vi "Drive Controller.vi"(8 "error in":errorcluster) -> ()   [LabVIEW 2020]
doc: "This VI executes continuously carrying out the current operation and responding to updates or new operation requests. It will often contain the timing or control code that is difficult to place directly in TeleOp. This VI generally opens all sensors and motors and isolates the rest of the robot code from knowing implementation details of how the operations are carried out."
uses:
  <vilib>/Rock Robotics/WPI/Framework/Completion Status.ctl
  Drive Setpoints.ctl
  Drive Operations.ctl
  <vilib>/Rock Robotics/WPI/SafetyOutput/WPI_SafetyOutputConfigMenu.ctl
  <vilib>/Rock Robotics/WPI/ThirdParty/REV Robotics/REVLib/Typedef/Spark MAX Motor Type.ctl
  <vilib>/Rock Robotics/WPI/ThirdParty/REV Robotics/REVLib/Typedef/Spark MAX Idle Mode.ctl
  <vilib>/Rock Robotics/WPI/RobotDrive/WPI_RobotDriveOpen2MotorWithExistingMotors.vi
  <vilib>/Rock Robotics/Network Tables/NT Write Numeric Array.vi
panel:
  in  "Interactive Values":T1
  in  "Buttons":cluster{"Execute Cmd":bool, "Abort Cmd":bool}
  out "Command Timing":cluster{"Start Time (ms)":u32, "Iterations":i32}
  out "Status":T3
  out "Setpoints":T4(graph)
  out "Current\nCmd":string
  # "Tip: The graph shows the motor setpoints. It may also be helpful to observe inputs and sensor values.\nYou may also want to display tuning or debugging controls."
  # "Interactive Command: You may fill in the settings for a command\nand schedule it with the Execute button. You can observe and abort\nany command while fine tuning the code for the controller."
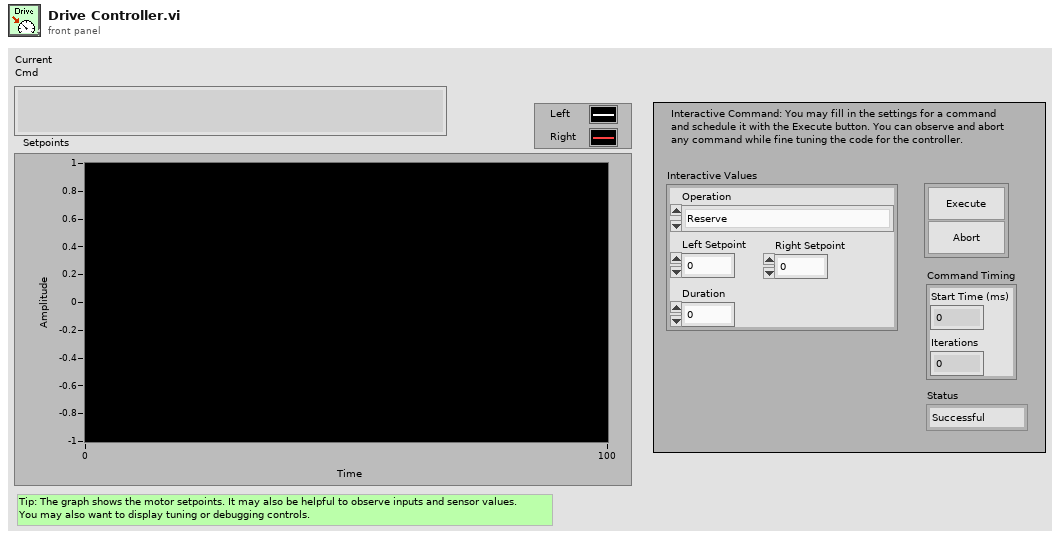
[diagram p1: front panel]
types:
  T1 = typedef "Drive Setpoints.ctl" = cluster{"Operation":T2, "Left Setpoint":dbl, "Right Setpoint":dbl, "Duration":dbl}
  T2 = typedef "Drive Operations.ctl" = enum16{"Reserve", "Read Current", "Immediate", "Drive for Time", "Drive for Distance"}
  T3 = typedef "Completion Status.ctl" = enum16{"Successful", "Aborted", "Incomplete"}
  T4 = cluster{"Left Setpoint":dbl, "Right Setpoint":dbl}
  T5 = typedef "Spark MAX Idle Mode.ctl" = enum16{"Coast", "Brake"}
  T6 = typedef "Spark MAX Motor Type.ctl" = enum16{"Brushed", "Brushless"}
  T7 = typedef "WPI_SafetyOutputConfigMenu.ctl" = enum16{"Enable", "Disable"}
  T8 = typedef "WPI_MotorControlDeviceRef.ctl" = cluster{"DeviceStatus":errorcluster, "Type":T9, "PWM":cluster{"PWM Channel":T10, "DeadBand":T11}, "CAN":cluster{"Device Number":u8, "SetOutput VI Ref":variant, "GetOutput VI Ref":variant, "Enable VI Ref":variant, "Disable VI Ref":variant, "Data":variant}, "Invert":bool, "DIO PWM":cluster{"PWM \"Enable\" Channel":T10, "DIOChannel":T12, "PWM Rate":dbl}}
  T9 = typedef "WPI_MotorControlType.ctl" = enum16{"PWM", "CAN", "DIO PWM"}
  T10 = typedef "FPGA_DIOPWMChannel.ctl" = enum8{"PWM 0", "PWM 1", "PWM 2", "PWM 3", "PWM 4", "PWM 5", "PWM 6", "PWM 7", "PWM 8", "PWM 9", "PWM MXP 0", "PWM MXP 1", "PWM MXP 2", "PWM MXP 3", "PWM MXP 4", "PWM MXP 5", "PWM MXP 6", "PWM MXP 7", "PWM MXP 8", "PWM MXP 9", "Invalid"}
  T11 = typedef "WPI_PWMDeadband.ctl" = cluster{"Name":string, "maxPositivePwm":i32, "minPositivePwm":i32, "centerPwm":i32, "maxNegativePwm":i32, "minNegativePwm":i32, "angularRange":u16}
  T12 = typedef "FPGA_DIOChannel.ctl" = enum8{"DIO 0", "DIO 1", "DIO 2", "DIO 3", "DIO 4", "DIO 5", "DIO 6", "DIO 7", "DIO 8", "DIO 9", "DIO MXP 0", "DIO MXP 1", "DIO MXP 2", "DIO MXP 3", "DIO MXP 4", "DIO MXP 5", "DIO MXP 6", "DIO MXP 7", "DIO MXP 8", "DIO MXP 9", "DIO MXP 10", "DIO MXP 11", "DIO MXP 12", "DIO MXP 13", "DIO MXP 14", "DIO MXP 15", "SPI Port CS1", "SPI Port CS2", "SPI Port CS3", "SPI Port MISO", "SPI Port MOSI", "Invalid"}
  T13 = typedef "WPI_RobotDriveDevRef.ctl" = cluster{"DevStatus":errorcluster, "Motors[]":T8[], "Square Inputs":bool, "Max Output":dbl}
  T14 = typedef "Command Status Info.ctl" = cluster{"Name":string, "Status":T3, "notifier out":T15}
  T15 = typedef "Completion Notifier.ctl" = refnum<notifier>
  T16 = cluster{"SubSystem Data":T1, cluster{"Start Time (ms)":u32, "Iterations":i32}, cluster{"Command Info":T14, "Description":string, "Default Command":T1, "queue out":refnum<queue>, "Subsystem Name":string}}
  T17 = cluster{"SubSystem Data":T1, cluster{"Start Time (ms)":u32, "Iterations":i32}, "Default Command Arguments":cluster{"Command Info":T14, "Description":string, "Default Command":T1, "queue out":refnum<queue>, "Subsystem Name":string}}
  T18 = cluster{"Don't move motors while reserved":dbl, "Don't move motors while reserved":dbl}
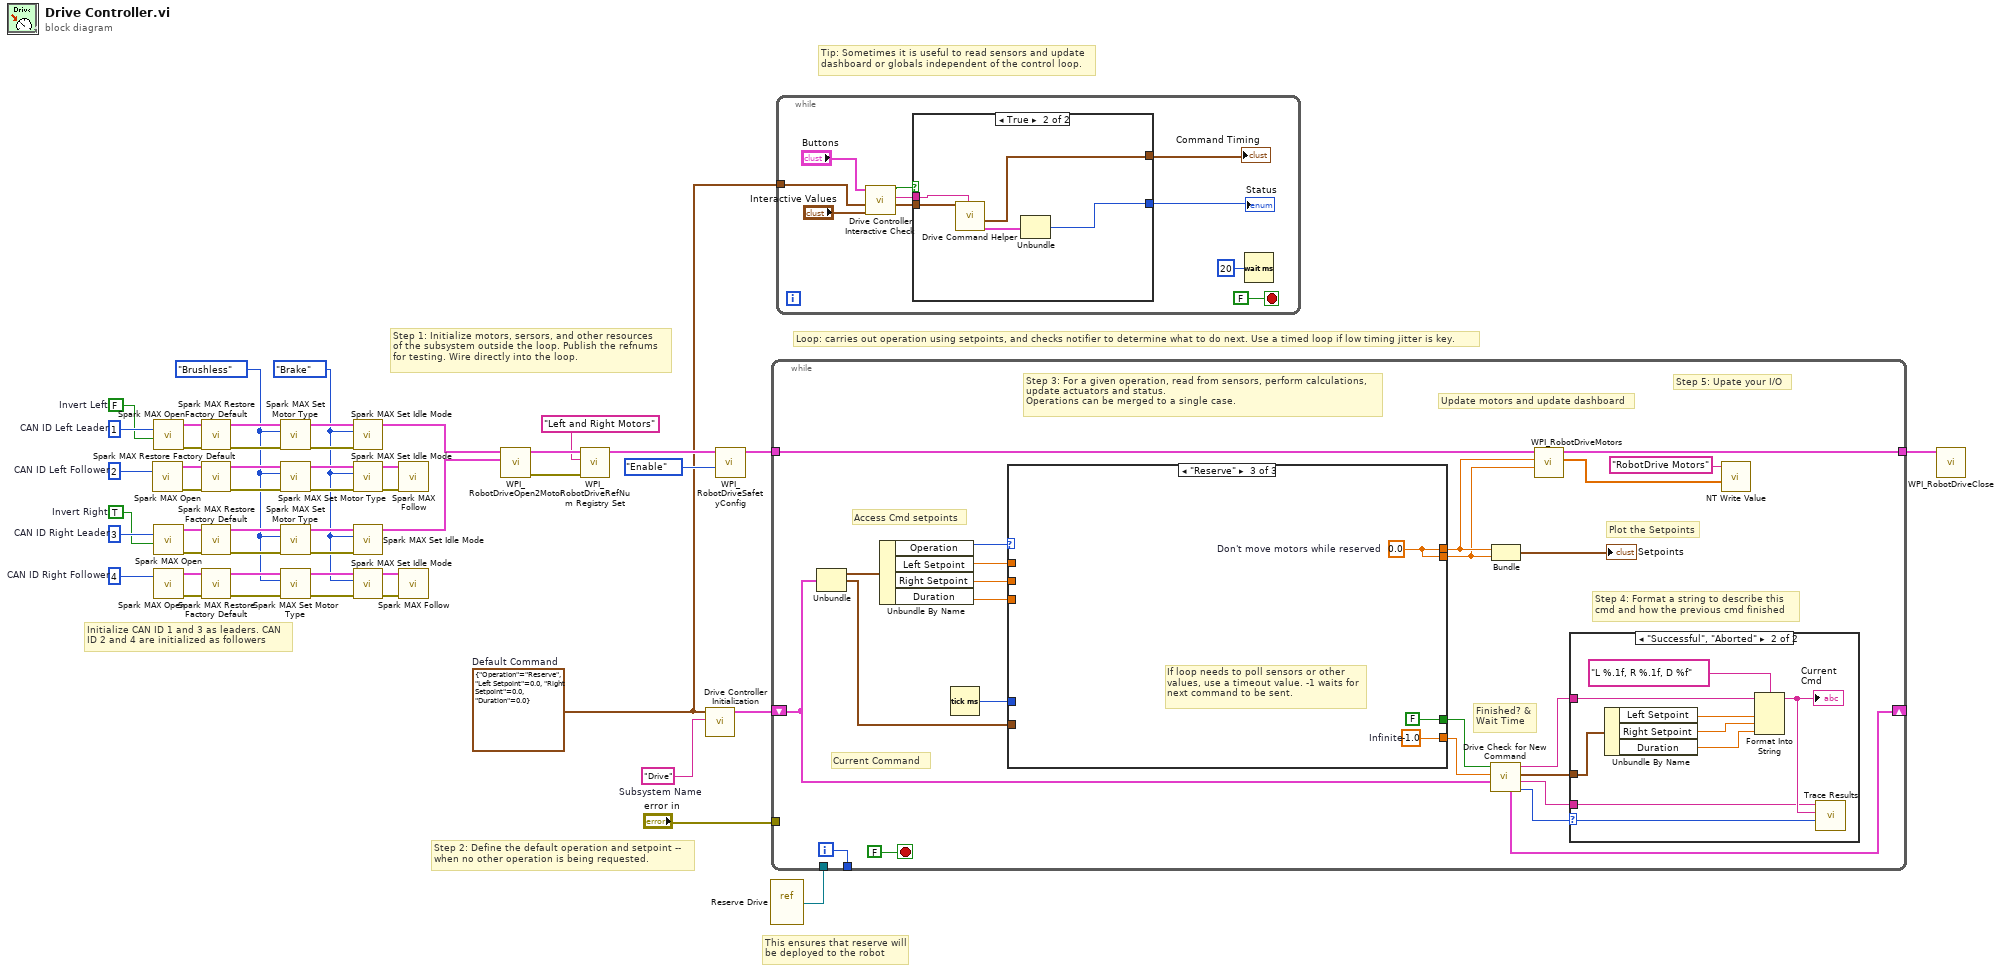
[diagram p0: block diagram]
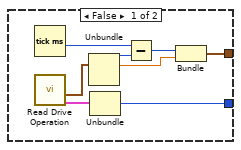
[diagram p2: hidden frame]
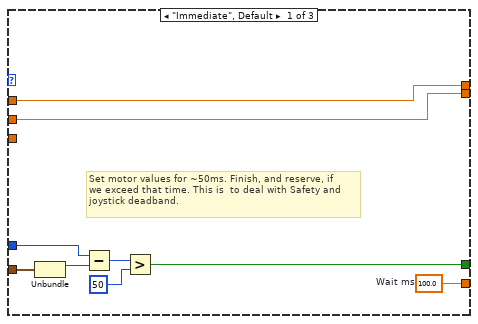
[diagram p4: hidden frame]
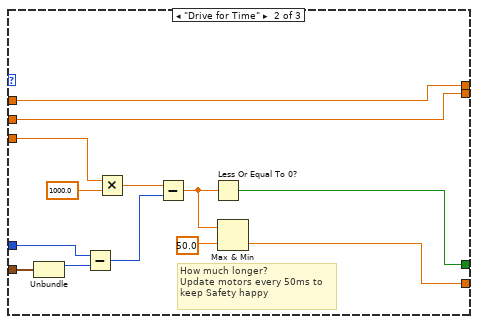
[diagram p5: hidden frame]
diagram:
  w8 = Spark_MAX_Idle_Mode."Brake" ("Idle Mode")
  w17 = Spark_MAX_Motor_Type."Brushless" ("Motor Type")
  w34 = FALSE  # Invert Left
  w35 = TRUE  # Invert Right
  w37 = u8 3  # CAN ID Right Leader
  w36 = u8 4  # CAN ID Right Follower
  w38 = u8 1  # CAN ID Left Leader
  w39 = u8 2  # CAN ID Left Follower
  w40 = T1 {"Operation"=enum."Reserve", "Left Setpoint"=0.0, "Right Setpoint"=0.0, "Duration"=0.0}  # Default Command
  w50 = "Drive"  # Subsystem Name
  # "Initialize CAN ID 1 and 3 as leaders. CAN \nID 2 and 4 are initialized as followers"
  # "This ensures that reserve will\nbe deployed to the robot"
  # "Tip: Sometimes it is useful to read sensors and update\ndashboard or globals independent of the control loop."
  # "Step 2: Define the default operation and setpoint --\nwhen no other operation is being requested."
  # "Step 1: Initialize motors, sersors, and other resources\nof the subsystem outside the loop. Publish the refnums\nfor testing. Wire directly into the loop."
  # "Loop: carries out operation using setpoints, and checks notifier to determine what to do next. Use a timed loop if low timing jitter is key."
  n1 = call <vilib>:"Spark MAX Open.vi"("Device Number"=w39) -> ("error out"=w31:errorcluster, "MotorControlDeviceRef"=w30:T8)  [unwired: 9 in]
  n2 = call <vilib>:"Spark MAX Open.vi"("Invert"=w34, "Device Number"=w38) -> ("error out"=w33:errorcluster, "MotorControlDeviceRef"=w32:T8)  [unwired: 8 in]
  n3 = call <vilib>:"Spark MAX Open.vi"("Invert"=w35, "Device Number"=w37) -> ("error out"=w29:errorcluster, "MotorControlDeviceRef"=w28:T8)  [unwired: 8 in]
  n4 = call <vilib>:"Spark MAX Open.vi"("Device Number"=w36) -> ("error out"=w27:errorcluster, "MotorControlDeviceRef"=w26:T8)  [unwired: 9 in]
  n5 = call <vilib>:"Spark MAX Restore Factory Default.vi"("error in"=w33, "MotorControlDeviceRef"=w32) -> ("error out"=w25:errorcluster, "MotorControlDeviceRef"=w24:T8)  [unwired: 8 in]
  n6 = call <vilib>:"Spark MAX Restore Factory Default.vi"("error in"=w31, "MotorControlDeviceRef"=w30) -> ("error out"=w23:errorcluster, "MotorControlDeviceRef"=w22:T8)  [unwired: 8 in]
  n7 = call <vilib>:"Spark MAX Restore Factory Default.vi"("error in"=w29, "MotorControlDeviceRef"=w28) -> ("error out"=w21:errorcluster, "MotorControlDeviceRef"=w20:T8)  [unwired: 8 in]
  n8 = call <vilib>:"Spark MAX Restore Factory Default.vi"("error in"=w27, "MotorControlDeviceRef"=w26) -> ("error out"=w19:errorcluster, "MotorControlDeviceRef"=w18:T8)  [unwired: 8 in]
  n9 = call <vilib>:"Spark MAX Set Motor Type.vi"("error in (no error)"=w25, "Motor Type"=w17, "MotorControlDevRef"=w24) -> ("error out"=w16:errorcluster, "MotorControlDeviceRef"=w15:T8)  [unwired: 7 in]
  n10 = call <vilib>:"Spark MAX Set Motor Type.vi"("error in (no error)"=w23, "Motor Type"=w17, "MotorControlDevRef"=w22) -> ("error out"=w14:errorcluster, "MotorControlDeviceRef"=w13:T8)  [unwired: 7 in]
  n11 = call <vilib>:"Spark MAX Set Motor Type.vi"("error in (no error)"=w21, "Motor Type"=w17, "MotorControlDevRef"=w20) -> ("error out"=w12:errorcluster, "MotorControlDeviceRef"=w11:T8)  [unwired: 7 in]
  n12 = call <vilib>:"Spark MAX Set Motor Type.vi"("error in (no error)"=w19, "Motor Type"=w17, "MotorControlDevRef"=w18) -> ("error out"=w10:errorcluster, "MotorControlDeviceRef"=w9:T8)  [unwired: 7 in]
  n13 = call <vilib>:"Spark MAX Set Idle Mode.vi"("error in (no error)"=w16, "Idle Mode"=w8, "MotorControlDeviceRef in"=w15) -> ("MotorControlDeviceRef out"=w3:T8)  [unwired: 7 in, 1 out]
  n14 = call <vilib>:"Spark MAX Set Idle Mode.vi"("error in (no error)"=w14, "Idle Mode"=w8, "MotorControlDeviceRef in"=w13) -> ("error out"=w7:errorcluster, "MotorControlDeviceRef out"=w6:T8)  [unwired: 7 in]
  n15 = call <vilib>:"Spark MAX Set Idle Mode.vi"("error in (no error)"=w12, "Idle Mode"=w8, "MotorControlDeviceRef in"=w11) -> ("MotorControlDeviceRef out"=w2:T8)  [unwired: 7 in, 1 out]
  n16 = call <vilib>:"Spark MAX Set Idle Mode.vi"("error in (no error)"=w10, "Idle Mode"=w8, "MotorControlDeviceRef in"=w9) -> ("error out"=w5:errorcluster, "MotorControlDeviceRef out"=w4:T8)  [unwired: 7 in]
  n17 = call <vilib>:"Spark MAX Follow.vi"("error in (no error)"=w7, "MotorControlDeviceRef"=w6) -> ()  [unwired: 8 in, 2 out]
  n18 = call <vilib>:"Spark MAX Follow.vi"("error in (no error)"=w5, "MotorControlDeviceRef"=w4) -> ()  [unwired: 8 in, 2 out]
  n19 = call-poly <vilib>:"WPI_RobotDriveOpen2Motor.vi"("Right Motor Dev Ref"=w2, "Left Motor Dev Ref"=w3) -> ("error out"=w47:errorcluster, "RobotDriveDevRef"=w49:T13)  [unwired: 3 in, 5 out]
  n20 = call <vilib>:"WPI_RobotDriveRefNum Registry Set.vi"("error in (no error)"=w47, "refnum name"="Left and Right Motors", "RobotDriveDevRef"=w49) -> ("RobotDriveDevRef"=w46:T13)  [unwired: 1 in, 7 out]
  n21 = call "Drive Controller Initialization.vi"("Subsystem Name"=w50, "Default Command"=w40) -> ("Current Command"=w42:T16)  [unwired: 9 in]
  n22 = call <vilib>:"WPI_RobotDriveSafetyConfig.vi"("mode"=WPI_SafetyOutputConfigMenu."Enable", "RobotDriveDevRef"=w46) -> ("RobotDriveDevRef"=w44:T13)  [unwired: 8 in, 1 out]
  n23 = vi-ref "Reserve Drive.vi"() -> (w41:refnum<vi>)
  n24 = while {
    shift-right: [w61] -> _
    shift-left: w42 -> [w54]
    tunnel: [w73] -> _
    tunnel: w44 -> [w69]
    tunnel: "error in" -> [_]
    tunnel: w41 -> [_]
    tunnel: [w53] -> w1
    i -> [w73]
    stop <- FALSE stop-if-true
    # "Step 5: Upate your I/O"
    # "Step 4: Format a string to describe this\ncmd and how the previous cmd finished"
    # "Current Command"
    # "Update motors and update dashboard"
    # "Plot the Setpoints"
    # "Access Cmd setpoints"
    # "Finished? &\nWait Time"
    # "Step 3: For a given operation, read from sensors, perform calculations,\nupdate actuators and status.\nOperations can be merged to a single case."
    n25 = Unbundle(w54) -> ("SubSystem Data"=w68:T1, w55:cluster{"Start Time (ms)":u32, "Iterations":i32})  [unwired: 1 out]
    n26 = Unbundle By Name(w68) -> ("Operation"=w67:T2, "Left Setpoint"=w66:dbl, "Right Setpoint"=w65:dbl, "Duration"=w64:dbl)
    n27 = Tick Count (ms)() -> (millisecond timer value=w63:u32)
    n28 = case shown="\"Reserve\"" w67 {
      tunnel: [w92 w93 w108] -> w60
      tunnel: [w85 w100 FALSE ("ignore previous (F)")] -> w59
      tunnel: w55 -> [w84 w102 _]
      tunnel: [w91 w99 w106] -> w71
      tunnel: [w90 w98 w106] -> w70
      tunnel: w66 -> [w91 w99 _]
      tunnel: w65 -> [w90 w98 _]
      tunnel: w64 -> [_ w97 _]
      tunnel: w63 -> [w86 w96 _]
      frame "Immediate", Default {
        w92 = 100.0  # Wait ms
        # "Set motor values for ~50ms. Finish, and reserve, if\nwe exceed that time. This is  to deal with Safety and\njoystick deadband."
        n29 = Unbundle(w84) -> ("Start Time (ms)"=w87:u32)  [unwired: 1 out]
        n30 = Subtract(x=w86, y=w87) -> (x-y=w88:u32)
        n31 = Greater?(x=w88, y=u8 50 ("Left Motor")) -> (0:w85:bool)
      }
      frame "Drive for Time" {
        # "How much longer?\nUpdate motors every 50ms to\nkeep Safety happy"
        n32 = Unbundle(w102) -> ("Start Time (ms)"=w101:u32)  [unwired: 1 out]
        n33 = Subtract(x=w96, y=w101) -> (x-y=w105:u32)
        n34 = Multiply(x=w97, y=1000.0) -> (x*y=w104:dbl)
        n35 = Subtract(x=w104, y=w105) -> (x-y=w95:dbl)
        n36 = Less Or Equal To 0?(x=w95) -> (x <= 0?=w100:bool)
        n37 = Max & Min(x=w95, y=50.0) -> (min(x,y)=w93:dbl)  [unwired: 1 out]
      }
      frame "Reserve" {
        w106 = 0.0  # Don't move motors while reserved
        w108 = -1.0  # Infinite
        # "If loop needs to poll sensors or other\nvalues, use a timeout value. -1 waits for\nnext command to be sent."
      }
    }
    n38 = call "Drive Check for New Command.vi"("input cluster"=w54, "Wait time (ms)"=w60, "Finished?"=w59) -> ("Completion"=w62:T3, "Subsystem Name"=w56:string, "Current Command"=w57:T1, "Initial Trace String"=w58:string, "Next Command"=w61:T17)  [unwired: 4 in]
    n39 = Bundle("Don't move motors while reserved"=w71, "Don't move motors while reserved"=w70) -> (→"Setpoints":T18)  [unwired: 1 in]
    n40 = call <vilib>:"WPI_RobotDriveMotors.vi"("RightSpeed"=w70, "LeftSpeed"=w71, "RobotDriveDevRef"=w69) -> ("Motor Values"=w52:dbl[], "RobotDriveDevRef"=w53:T13)  [unwired: 1 in, 6 out]
    n41 = case shown="\"Successful\", \"Aborted\"" w62 {
      selector: w62 -> [_ w83]
      tunnel: w58 -> [_ w78]
      tunnel: w57 -> [_ w79]
      tunnel: w56 -> [_ w75]
      frame "Incomplete", Default {
        # "Continuing current command"
      }
      frame "Successful", "Aborted" {
        # "Report and setup for next command"
        n42 = Unbundle By Name(w79) -> ("Left Setpoint"=w81:dbl, "Right Setpoint"=w82:dbl, "Duration"=w76:dbl)
        n43 = Format Into String(format string="L %.1f, R %.1f, D %f", initial string=w78, w81, w82, w76) -> (resulting string=w77:string)  [unwired: 1 in, 1 out]
        "Current\nCmd" <- w77
        n44 = call <vilib>:"Trace Results.vi"("Status of previous command"=w83, "Description"=w77, "Subsystem"=w75) -> ()  [unwired: 9 in]
      }
    }
    n45 = call-poly <vilib>:"NT Write Value.vi"("Numeric Array"=w52, "Name"="RobotDrive Motors") -> ()  [unwired: 9 in, 1 out]
  }
  n46 = while {
    tunnel: w40 -> [w110]
    stop <- FALSE stop-if-true
    n47 = call "Drive Controller Interactive Check.vi"("Interactive Command In"="Interactive Values", "Default Command"=w110, "Buttons"="Buttons") -> ("Interactive Command Out"=w112:T1, "Trace String"=w113:string, "Schedule"=w114:bool)  [unwired: 6 in]
    n48 = case shown="True" w114 {
      tunnel: [w123 w131] -> w115
      tunnel: [w122 w127] -> w116
      tunnel: w113 -> [_ w129]
      tunnel: w112 -> [_ w128]
      frame False {
        n49 = Tick Count (ms)() -> (millisecond timer value=w126:u32)
        n50 = call "Read Drive Operation.vi"() -> ("Command Info"=w120:T14, "SubSystem Data"=w119:T1)  [unwired: 9 in, 1 out]
        n51 = Unbundle(w119) -> ("Operation"=w124:T2, "Left Setpoint"=w121:dbl)  [unwired: 2 out]
        n52 = Unbundle(w120) -> ("Status"=w123:T3)  [unwired: 2 out]
        n53 = Subtract(x=w126, y=w124) -> (x-y=w125:u32)
        n54 = Bundle(w125, "Left Setpoint"=w121) -> (w122:cluster{u32, "Left Setpoint":dbl})  [unwired: 1 in]
      }
      frame True {
        n55 = call "Drive Command Helper.vi"("Description"=w129, "SubSystem Data"=w128) -> ("Command Info Out"=w130:T14, "Command Timing"=w127:cluster{"Start Time (ms)":u32, "Iterations":i32})  [unwired: 7 in, 1 out]
        n56 = Unbundle(w130) -> ("Status"=w131:T3)  [unwired: 2 out]
      }
    }
    "Status" <- w115
    "Command Timing" <- w116
    n57 = Wait (ms)(milliseconds to wait=u32 20) -> ()  [unwired: 1 out]
  }
  n58 = call <vilib>:"WPI_RobotDriveClose.vi"("RobotDriveDevRef"=w1) -> ()  [unwired: 10 in, 1 out]
